vi "LaunchService.vi"(8 "error in (no error)":errorcluster, 11 "Service Details Out":T1) -> (0 "error out":errorcluster, 3 "Default Connection String":string)   [LabVIEW 2019, in "MicronClient.lvclass"]
uses:
  MicronClient.lvclass
  <vilib>/SLL Toolkit/SLL String/SLL String.lvlib
  <vilib>/SLL Toolkit/SLL String/_SubVIs/1D String Array to String.vi
  Typedefs/ServiceDetails.ctl
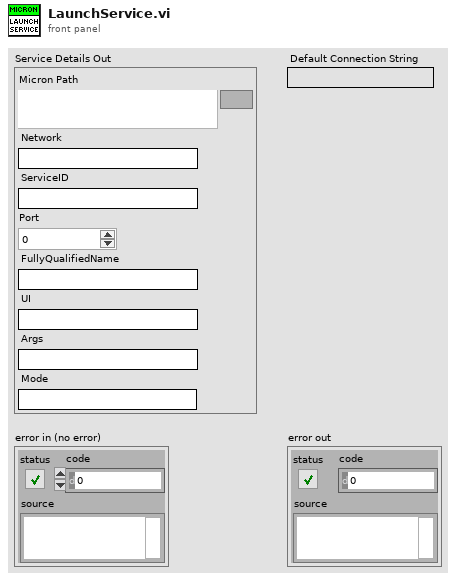
[diagram p1: front panel]
types:
  T1 = typedef "MicronClient.lvclass/ServiceDetails.ctl" = cluster{"Micron Path":path, "Network":string, "ServiceID":string, "Port":i32, "FullyQualifiedName":string, "UI":string, "Args":string, "Mode":string}
  T2 = typedef "MicronClient.lvclass/MicronModeINISection.ctl" = cluster{"Command":string, "WorkingDirectory":path}
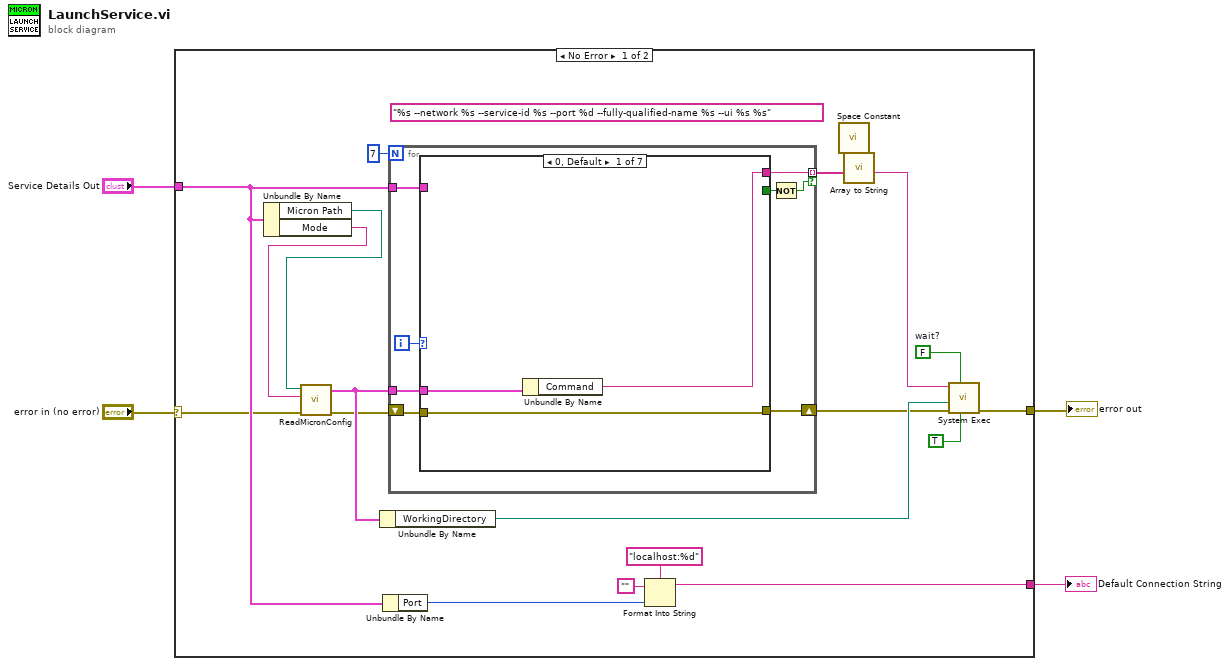
[diagram p0: block diagram]
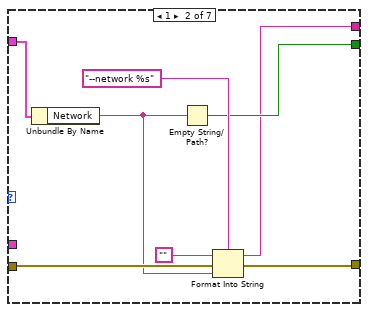
[diagram p2: hidden frame]
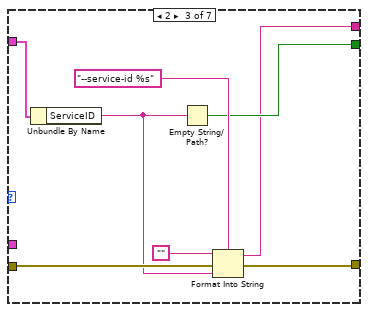
[diagram p3: hidden frame]
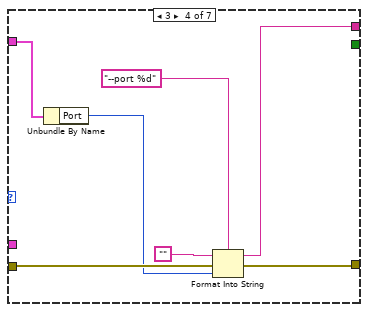
[diagram p4: hidden frame]
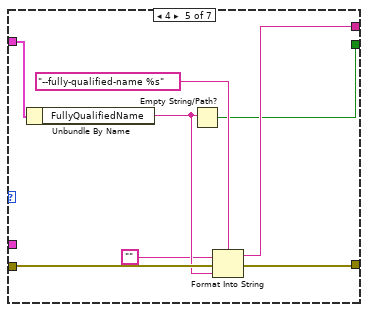
[diagram p5: hidden frame]
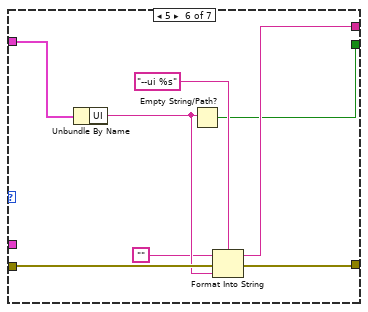
[diagram p6: hidden frame]
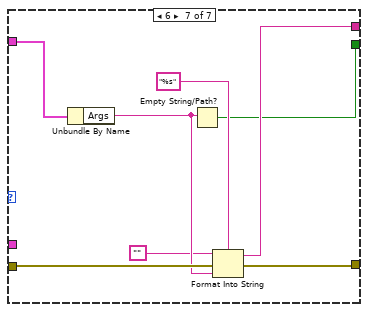
[diagram p7: hidden frame]
diagram:
  n1 = case shown="No Error" "error in (no error)" {
    selector: "error in (no error)" -> [w17 w82]
    tunnel: "Service Details Out" -> [w19 _]
    tunnel: [w15 _] -> w2
    tunnel: [w13 w82] -> w1
    frame No Error {
      (unwired) "%s --network %s --service-id %s --port %d --fully-qualified-name %s --ui %s %s" ("format string")
      w5 = FALSE  # wait?
      n2 = Unbundle By Name(w19) -> ("Micron Path"=w20:path, "Mode"=w23:string)
      n3 = call "ReadMicronConfig.vi"("Error In"=w17, "Mode"=w23, "Micron Path In"=w20) -> ("Error Out"=w18:errorcluster, "Micron Mode"=w21:T2)  [unwired: 7 in]
      n4 = Unbundle By Name(w21) -> ("WorkingDirectory"=w22:path)
      n5 = Unbundle By Name(w19) -> ("Port"=w14:i32)
      n6 = for {
        N: 7 -> [_]
        tunnel: w19 -> [w30]
        shift-right: [w28] -> w6
        shift-left: w18 -> [w29]
        tunnel: [w27] -> w10 mode=indexing if=w25
        tunnel: w21 -> [w24]
        i -> [w31]
        n7 = case shown="0, Default" w31 {
          tunnel: w30 -> [_ w42 w50 w57 w65 w73 w81]
          tunnel: w29 -> [w32 w41 w49 w56 w64 w72 w80]
          tunnel: [w32 w40 w48 w55 w63 w71 w79] -> w28
          tunnel: [w34 w36 w44 w52 w61 w69 w77] -> w27
          tunnel: [_ w37 w45 _ w59 w67 w75] -> w26
          tunnel: w24 -> [w33 _ _ _ _ _ _]
          frame 0, Default {
            n8 = Unbundle By Name(w33) -> ("Command"=w34:string)
          }
          frame 1 {
            n9 = Unbundle By Name(w42) -> ("Network"=w38:string)
            n10 = Empty String/Path?(string/path=w38) -> (empty?=w37:bool)
            n11 = Format Into String(format string="--network %s", initial string="", error in=w41, w38) -> (resulting string=w36:string, error out=w40:errorcluster)
          }
          frame 2 {
            n12 = Unbundle By Name(w50) -> ("ServiceID"=w46:string)
            n13 = Empty String/Path?(string/path=w46) -> (empty?=w45:bool)
            n14 = Format Into String(format string="--service-id %s", initial string="", error in=w49, w46) -> (resulting string=w44:string, error out=w48:errorcluster)
          }
          frame 3 {
            n15 = Unbundle By Name(w57) -> ("Port"=w53:i32)
            n16 = Format Into String(format string="--port %d", initial string="", error in=w56, w53) -> (resulting string=w52:string, error out=w55:errorcluster)
          }
          frame 4 {
            n17 = Unbundle By Name(w65) -> ("FullyQualifiedName"=w60:string)
            n18 = Empty String/Path?(string/path=w60) -> (empty?=w59:bool)
            n19 = Format Into String(format string="--fully-qualified-name %s", initial string="", error in=w64, w60) -> (resulting string=w61:string, error out=w63:errorcluster)
          }
          frame 5 {
            n20 = Unbundle By Name(w73) -> ("UI"=w68:string)
            n21 = Empty String/Path?(string/path=w68) -> (empty?=w67:bool)
            n22 = Format Into String(format string="--ui %s", initial string="", error in=w72, w68) -> (resulting string=w69:string, error out=w71:errorcluster)
          }
          frame 6 {
            n23 = Unbundle By Name(w81) -> ("Args"=w76:string)
            n24 = Empty String/Path?(string/path=w76) -> (empty?=w75:bool)
            n25 = Format Into String(format string="%s", initial string="", error in=w80, w76) -> (resulting string=w77:string, error out=w79:errorcluster)
          }
        }
        n26 = Not(x=w26) -> (.not. x?=w25:bool)
      }
      n27 = Format Into String(format string="localhost:%d", initial string="", w14) -> (resulting string=w15:string)  [unwired: 1 in, 1 out]
      n28 = call <vilib>:"Space Constant.vi"() -> ("String"=w11:string)
      n29 = call-poly <vilib>:"Array to String.vi"("Delimiter (,)"=w11, "1D Array[]"=w10) -> ("String"=w7:string)  [unwired: 6 in]
      n30 = call <vilib>:"System Exec.vi"("run minimized? (F)"=TRUE, "wait until completion? (T)"=w5, "error in (no error)"=w6, "working directory"=w22, "command line"=w7) -> ("error out"=w13:errorcluster)  [unwired: 3 in, 3 out]
    }
    frame Error {
    }
  }
  "Default Connection String" <- w2
  "error out" <- w1
